vi "Find_Rows_to_Combine.vi"(4 "Include Empty Rows?":bool, 5 "file path (dialog if empty)":path, 6 "Give Audit Channels":bool, 7 "Full Channel Names":string[](array[string]), 8 "Data":string[][](array[string]), 9 "Z Column Index":i32, 10 "Y Column Index":i32, 11 "X Column Index":i32) -> ()   [LabVIEW 2020]
uses:
  Results_plotter_Global.vi
panel:
  in  "Case Constant\n(See Context Help)":i32=1
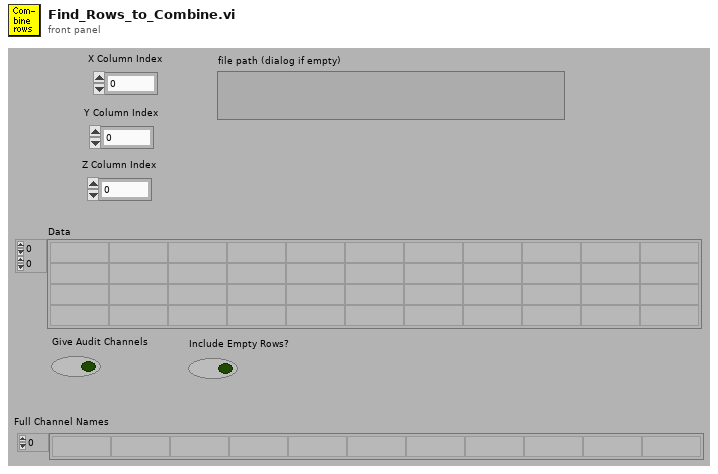
[diagram p1: front panel]
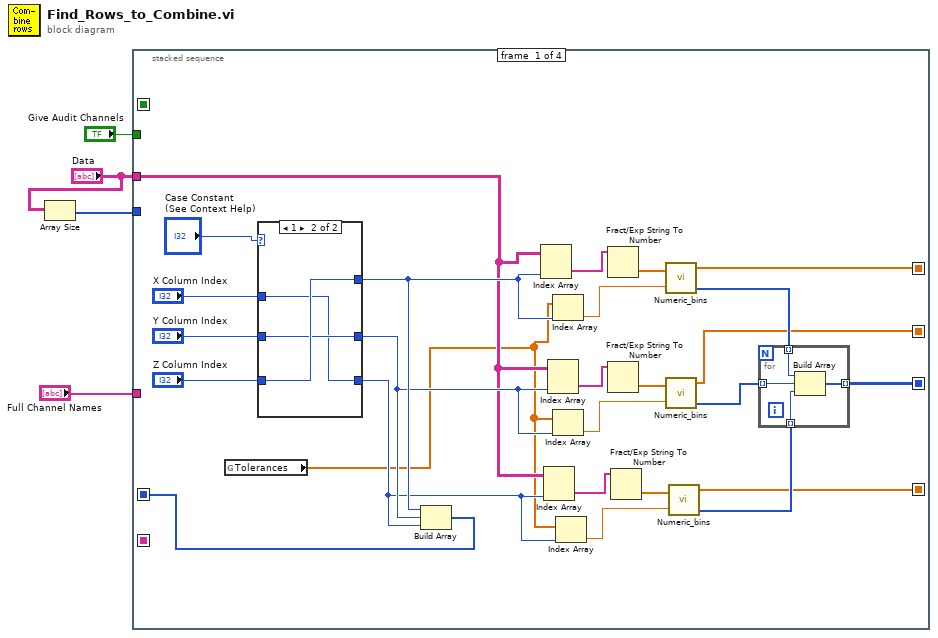
[diagram p0: block diagram]
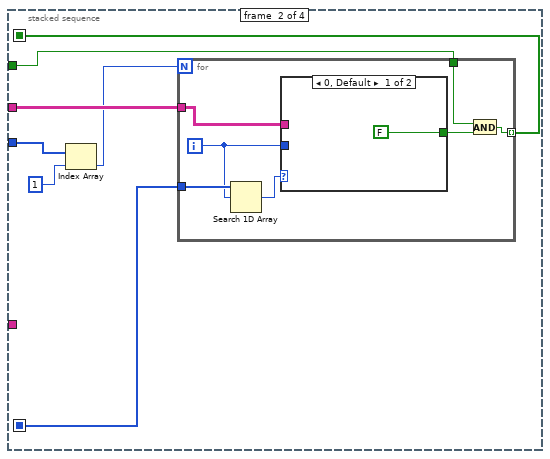
[diagram p3: hidden frame]
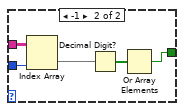
[diagram p4: hidden frame]
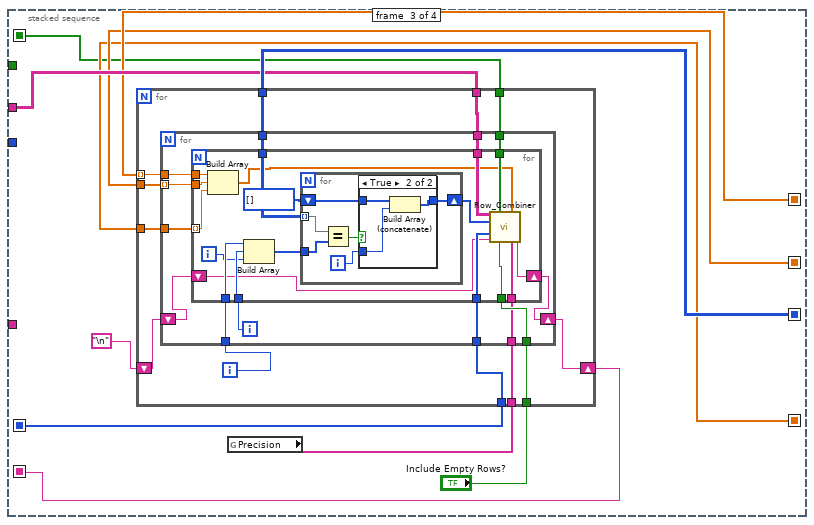
[diagram p5: hidden frame]
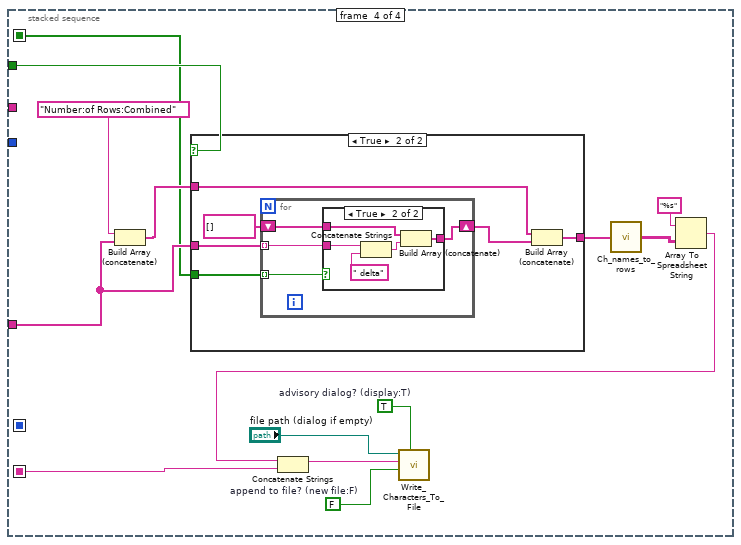
[diagram p7: hidden frame]
diagram:
  n1 = Array Size(array="Data") -> (size(s)=w1:i32[])
  n2 = stacked-sequence {
    seq-local: [w10 _ _ _] -> [_ w43 w64 _]
    seq-local: [w9 _ _ _] -> [_ _ w67 _]
    seq-local: [w8 _ _ _] -> [_ _ w66 _]
    seq-local: [w6 _ _ _] -> [_ _ w65 _]
    seq-local: [w7 _ _ _] -> [_ _ w69 _]
    seq-local: [_ _ w63 _] -> [_ _ _ w130]
    seq-local: [_ w42 _ _] -> [_ _ w62 w125]
    tunnel: "Data" -> [w11 w45 w68 _]
    tunnel: "Give Audit Channels" -> [_ w41 _ w137]
    tunnel: "Full Channel Names" -> [_ _ _ w136]
    tunnel: w1 -> [_ w46 _ _]
    frame #0 {
      n3 = global read "Results_plotter_Global.vi" "Tolerances"() -> (w5:dbl[])
      n4 = case shown="1" "Case Constant\n(See Context Help)" {
        tunnel: [w37 w40] -> w14
        tunnel: "X Column Index" -> [w37 w38]
        tunnel: [w36 w39] -> w13
        tunnel: "Y Column Index" -> [w36 w39]
        tunnel: [w35 w38] -> w12
        tunnel: "Z Column Index" -> [w35 w40]
        frame 0, Default {
        }
        frame 1 {
        }
      }
      n5 = Build Array(w14, w13, w12) -> (w10:i32[])
      n6 = Index Array(array=w11, index (col)=w14) -> (element=w30:string[])  [unwired: 1 in]
      n7 = Index Array(array=w11, index (col)=w12) -> (element=w23:string[])  [unwired: 1 in]
      n8 = Index Array(array=w11, index (col)=w13) -> (element=w24:string[])  [unwired: 1 in]
      n9 = Index Array(array=w5, index=w14) -> (element=w28:dbl)
      n10 = Index Array(array=w5, index=w13) -> (element=w26:dbl)
      n11 = Index Array(array=w5, index=w12) -> (element=w21:dbl)
      n12 = Fract/Exp String To Number(string=w30) -> (number=w29:dbl[])  [unwired: 4 out]
      n13 = Fract/Exp String To Number(string=w24) -> (number=w25:dbl[])  [unwired: 4 out]
      n14 = Fract/Exp String To Number(string=w23) -> (number=w22:dbl[])  [unwired: 4 out]
      n15 = call "Numeric_bins.vi"("Values"=w29, "Tolerance"=w28) -> ("Bin Centres"=w9:dbl[], "Bin Index"=w20:i32[])  [unwired: 1 out]
      n16 = call "Numeric_bins.vi"("Values"=w25, "Tolerance"=w26) -> ("Bin Centres"=w8:dbl[], "Bin Index"=w19:i32[])  [unwired: 1 out]
      n17 = call "Numeric_bins.vi"("Values"=w22, "Tolerance"=w21) -> ("Bin Centres"=w6:dbl[], "Bin Index"=w18:i32[])  [unwired: 1 out]
      n18 = for {
        tunnel: w20 -> [w34] mode=indexing
        tunnel: w19 -> [w33] mode=indexing
        tunnel: w18 -> [w32] mode=indexing
        tunnel: [w31] -> w7 mode=indexing
        n19 = Build Array(w34, w33, w32) -> (w31:i32[])
      }
    }
    frame #1 {
      n20 = Index Array(array=w46, index=1) -> (element=w44:i32)
      n21 = for {
        N: w44 -> [_]
        tunnel: w45 -> [w54]
        tunnel: w43 -> [w53]
        tunnel: [w49] -> w42 mode=indexing
        tunnel: w41 -> [w48]
        i -> [w52]
        n22 = Search 1D Array(1D array=w53, element=w52) -> (index of element=w51:i32)  [unwired: 1 out]
        n23 = case shown="0, Default" w51 {
          tunnel: w54 -> [_ w60]
          tunnel: w52 -> [_ w57]
          tunnel: [FALSE w56] -> w50
          frame 0, Default {
          }
          frame -1 {
            n24 = Index Array(array=w60, index (col)=w57) -> (element=w59:string[])  [unwired: 1 in]
            n25 = Decimal Digit?(1:w59) -> (0:w58:bool[])
            n26 = Or Array Elements(Boolean array=w58) -> (logical OR=w56:bool)
          }
        }
        n27 = And(x=w48, y=w50) -> (x .and. y?=w49:bool)
      }
    }
    frame #2 {
      n28 = global read "Results_plotter_Global.vi" "Precision"() -> (w71:string[])
      n29 = for {
        tunnel: w69 -> [w83]
        tunnel: w68 -> [w81]
        tunnel: w64 -> [w80]
        shift-right: [w78] -> w63
        shift-left: "\n" -> [w79]
        tunnel: "Include Empty Rows?" -> [w77]
        tunnel: w67 -> [w76] mode=indexing
        tunnel: w66 -> [w75]
        tunnel: w65 -> [w74]
        tunnel: w62 -> [w73]
        tunnel: w71 -> [w72]
        i -> [w82]
        n30 = for {
          tunnel: w83 -> [w96]
          tunnel: w82 -> [w95]
          tunnel: w81 -> [w93]
          tunnel: w80 -> [w92]
          shift-right: [w90] -> w78
          shift-left: w79 -> [w91]
          tunnel: w77 -> [w89]
          tunnel: w76 -> [w88]
          tunnel: w75 -> [w87] mode=indexing
          tunnel: w74 -> [w86]
          tunnel: w73 -> [w85]
          tunnel: w72 -> [w84]
          i -> [w94]
          n31 = for {
            tunnel: w96 -> [w114]
            tunnel: w95 -> [w111]
            tunnel: w94 -> [w110]
            tunnel: w93 -> [w109]
            tunnel: w92 -> [w105]
            shift-right: [w103] -> w90
            shift-left: w91 -> [w104]
            tunnel: w89 -> [w106]
            tunnel: w88 -> [w102]
            tunnel: w87 -> [w101]
            tunnel: w86 -> [w100] mode=indexing
            tunnel: w85 -> [w99]
            tunnel: w84 -> [w97]
            i -> [w107]
            n32 = Build Array(w102, w101, w100) -> (w98:dbl[])
            n33 = Build Array(w111, w110, w107) -> (w113:i32[])
            n34 = for {
              tunnel: w114 -> [w120] mode=indexing
              tunnel: w113 -> [w119]
              shift-right: [w115] -> w108
              shift-left: i32[] [] -> [w117]
              i -> [w116]
              n35 = Equal?(x=w120, y=w119) -> (x = y?=w118:bool)
              n36 = case shown="True" w118 {
                tunnel: w117 -> [w121 w124]
                tunnel: w116 -> [_ w123]
                tunnel: [w121 w122] -> w115
                frame False {
                }
                frame True {
                  n37 = Build Array (concatenate)(w124, w123) -> (w122:i32[])
                }
              }
            }
            n38 = call "Row_Combiner.vi"("All Data"=w109, "Audit Channels"=w99, "Coordinates"=w98, "Rows to Combine"=w108, "Position Columns"=w105, "String In"=w104, "Include Empty Rows?"=w106, "Precision"=w97) -> ("String Out"=w103:string)  [unwired: 7 out]
          }
        }
      }
    }
    frame #3 {
      w126 = TRUE  # advisory dialog? (display:T)
      w127 = FALSE  # append to file? (new file:F)
      n39 = Build Array (concatenate)("Number:of Rows:Combined", w136) -> (w135:string[])
      n40 = case shown="True" w137 {
        tunnel: w136 -> [_ w145]
        tunnel: w135 -> [w139 w144]
        tunnel: [w139 w143] -> w133
        tunnel: w125 -> [_ w140]
        frame False {
        }
        frame True {
          n41 = for {
            tunnel: w145 -> [w149] mode=indexing
            shift-right: [w147] -> w141
            shift-left: string[] [] -> [w148]
            tunnel: w140 -> [w146] mode=indexing
            n42 = case shown="True" w146 {
              tunnel: w149 -> [_ w155]
              tunnel: w148 -> [w150 w152]
              tunnel: [w150 w151] -> w147
              frame False {
              }
              frame True {
                n43 = Concatenate Strings(w155, " delta" ("string")) -> (w153:string)
                n44 = Build Array (concatenate)(w152, w153) -> (w151:string[])
              }
            }
          }
          n45 = Build Array (concatenate)(w144, w141) -> (w143:string[])
        }
      }
      n46 = call "Ch_names_to_rows.vi"("Channel Names"=w133) -> ("3 Row names"=w132:string[][])
      n47 = Array To Spreadsheet String(array=w132, 3:"%s" ("format string")) -> (spreadsheet string=w131:string)  [unwired: 1 out]
      n48 = Concatenate Strings(w131, w130) -> (w129:string)
      n49 = call "Write_Characters_To_File.vi"("file path (dialog if empty)"="file path (dialog if empty)", "advisory dialog? (display:T)"=w126, "character string"=w129, "append to file? (new file:F)"=w127) -> ()  [unwired: 1 in, 4 out]
    }
  }
